vi "Read_Write_Plot_Setup.vi"(2 "Mode":enum16{"Load", "Save"}(ring), 3 "Setup filename":string, 4 "Cluster":T1={"Result files to read"=[], "Template"=path "", "Transpose"=FALSE, "Additional X Values"=[], "Additional Y Values"=[], "Ordinate"=0, "Absisca"=0, "Filter Array"=[0, 0, 0, 0, 0, 0], "color and symbol"=FALSE, "Output Filename"=path "", "Jpg Vi Name"="Intensity plot jpg.vi", "Intensity Plot?"=FALSE, "Multi Ordinate?"=FALSE, "Filter Bins 1"=[0], "Filter Bins 2"=[0], "Multi Ordinate"=[]} {"Filter Array" items=["Don't Filter", "Measurement Type", "Seconds Since 1904", "X [mm]", "Y [mm]", "Z [mm]", "U [ms-1] Raw", "U [ms-1]", "U/Uref", "V [ms-1]", "V/Uref", "W [ms-1]", "W/Uref", "u^2 [m2s-2] Raw", "u^2 [m2s-2]", "u^2/Ur^2", "v^2 [m2s-2] Raw", "v^2 [m2s-2]", "v^2/Ur^2", "w^2 [m2s-2] Raw", "w^2 [m2s-2]", "w^2/Ur^2", "uv [m2s-2] Raw", "uv [m2s-2]", "uv/Ur^2", "uw [m2s-2] Raw", "uw [m2s-2]", "uw/Ur^2", "Average Sampling Rate [Hz]", "Flow Measurement Time [mins]", "Tunnel Velocity Uref [ms-1]", "Measurement Record Date", "Measurement Record Time", "Original Results Folder", "Original Results Filename", "Original Results Raw Data File", "Comments", "Roughness Pattern", "Roughness Element", "Roughness Element Height (mm)", "Roughness Unit size", "Roughness Area Density (%)", "Roughness Elements In a Unit", "Roughness Baseboard Vertical Displacement (mm)", "A Tunnel Metadata Travers Origin X Offset", "XW Angle Psi 1", "XW Angle Psi 2", "Tutu & Chevray Error in uw Correlation", "XW (UW) Calibration Drift", "Reference Temperature Deg C"]; "Absisca" items=["Measurement Type", "Seconds Since 1904", "X [mm]", "Y [mm]", "Z [mm]", "U [ms-1] Raw", "U [ms-1]", "U/Uref", "V [ms-1]", "V/Uref", "W [ms-1]", "W/Uref", "u^2 [m2s-2] Raw", "u^2 [m2s-2]", "u^2/Ur^2", "v^2 [m2s-2] Raw", "v^2 [m2s-2]", "v^2/Ur^2", "w^2 [m2s-2] Raw", "w^2 [m2s-2]", "w^2/Ur^2", "uv [m2s-2] Raw", "uv [m2s-2]", "uv/Ur^2", "uw [m2s-2] Raw", "uw [m2s-2]", "uw/Ur^2", "Average Sampling Rate [Hz]", "Flow Measurement Time [mins]", "Tunnel Velocity Uref [ms-1]", "Measurement Record Date", "Measurement Record Time", "Original Results Folder", "Original Results Filename", "Original Results Raw Data File", "Comments", "Roughness Pattern", "Roughness Element", "Roughness Element Height (mm)", "Roughness Unit size", "Roughness Area Density (%)", "Roughness Elements In a Unit", "Roughness Baseboard Vertical Displacement (mm)", "A Tunnel Metadata Travers Origin X Offset", "XW Angle Psi 1", "XW Angle Psi 2", "Tutu & Chevray Error in uw Correlation", "XW (UW) Calibration Drift", "Reference Temperature Deg C"]; "Ordinate" items=["Measurement Type", "Seconds Since 1904", "X [mm]", "Y [mm]", "Z [mm]", "U [ms-1] Raw", "U [ms-1]", "U/Uref", "V [ms-1]", "V/Uref", "W [ms-1]", "W/Uref", "u^2 [m2s-2] Raw", "u^2 [m2s-2]", "u^2/Ur^2", "v^2 [m2s-2] Raw", "v^2 [m2s-2]", "v^2/Ur^2", "w^2 [m2s-2] Raw", "w^2 [m2s-2]", "w^2/Ur^2", "uv [m2s-2] Raw", "uv [m2s-2]", "uv/Ur^2", "uw [m2s-2] Raw", "uw [m2s-2]", "uw/Ur^2", "Average Sampling Rate [Hz]", "Flow Measurement Time [mins]", "Tunnel Velocity Uref [ms-1]", "Measurement Record Date", "Measurement Record Time", "Original Results Folder", "Original Results Filename", "Original Results Raw Data File", "Comments", "Roughness Pattern", "Roughness Element", "Roughness Element Height (mm)", "Roughness Unit size", "Roughness Area Density (%)", "Roughness Elements In a Unit", "Roughness Baseboard Vertical Displacement (mm)", "A Tunnel Metadata Travers Origin X Offset", "XW Angle Psi 1", "XW Angle Psi 2", "Tutu & Chevray Error in uw Correlation", "XW (UW) Calibration Drift", "Reference Temperature Deg C"]; "Additional Y Values" format="%.2f"; "Additional X Values" format="%.2f"}) -> (0 "OK?":bool, 1 "Cluster 2":T1={"Result files to read"=[], "Template"=path "", "Transpose"=FALSE, "Additional X Values"=[], "Additional Y Values"=[], "Ordinate"=0, "Absisca"=0, "Filter Array"=[0, 0, 0, 0, 0, 0], "color and symbol"=FALSE, "Output Filename"=path "", "Jpg Vi Name"="Intensity plot jpg.vi", "Intensity Plot?"=FALSE, "Multi Ordinate?"=FALSE, "Filter Bins 1"=[0], "Filter Bins 2"=[0], "Multi Ordinate"=[]} {"Filter Array" items=["Don't Filter", "Measurement Type", "Seconds Since 1904", "X [mm]", "Y [mm]", "Z [mm]", "U [ms-1] Raw", "U [ms-1]", "U/Uref", "V [ms-1]", "V/Uref", "W [ms-1]", "W/Uref", "u^2 [m2s-2] Raw", "u^2 [m2s-2]", "u^2/Ur^2", "v^2 [m2s-2] Raw", "v^2 [m2s-2]", "v^2/Ur^2", "w^2 [m2s-2] Raw", "w^2 [m2s-2]", "w^2/Ur^2", "uv [m2s-2] Raw", "uv [m2s-2]", "uv/Ur^2", "uw [m2s-2] Raw", "uw [m2s-2]", "uw/Ur^2", "Average Sampling Rate [Hz]", "Flow Measurement Time [mins]", "Tunnel Velocity Uref [ms-1]", "Measurement Record Date", "Measurement Record Time", "Original Results Folder", "Original Results Filename", "Original Results Raw Data File", "Comments", "Roughness Pattern", "Roughness Element", "Roughness Element Height (mm)", "Roughness Unit size", "Roughness Area Density (%)", "Roughness Elements In a Unit", "Roughness Baseboard Vertical Displacement (mm)", "A Tunnel Metadata Travers Origin X Offset", "XW Angle Psi 1", "XW Angle Psi 2", "Tutu & Chevray Error in uw Correlation", "XW (UW) Calibration Drift", "Reference Temperature Deg C"]; "Absisca" items=["Measurement Type", "Seconds Since 1904", "X [mm]", "Y [mm]", "Z [mm]", "U [ms-1] Raw", "U [ms-1]", "U/Uref", "V [ms-1]", "V/Uref", "W [ms-1]", "W/Uref", "u^2 [m2s-2] Raw", "u^2 [m2s-2]", "u^2/Ur^2", "v^2 [m2s-2] Raw", "v^2 [m2s-2]", "v^2/Ur^2", "w^2 [m2s-2] Raw", "w^2 [m2s-2]", "w^2/Ur^2", "uv [m2s-2] Raw", "uv [m2s-2]", "uv/Ur^2", "uw [m2s-2] Raw", "uw [m2s-2]", "uw/Ur^2", "Average Sampling Rate [Hz]", "Flow Measurement Time [mins]", "Tunnel Velocity Uref [ms-1]", "Measurement Record Date", "Measurement Record Time", "Original Results Folder", "Original Results Filename", "Original Results Raw Data File", "Comments", "Roughness Pattern", "Roughness Element", "Roughness Element Height (mm)", "Roughness Unit size", "Roughness Area Density (%)", "Roughness Elements In a Unit", "Roughness Baseboard Vertical Displacement (mm)", "A Tunnel Metadata Travers Origin X Offset", "XW Angle Psi 1", "XW Angle Psi 2", "Tutu & Chevray Error in uw Correlation", "XW (UW) Calibration Drift", "Reference Temperature Deg C"]; "Ordinate" items=["Measurement Type", "Seconds Since 1904", "X [mm]", "Y [mm]", "Z [mm]", "U [ms-1] Raw", "U [ms-1]", "U/Uref", "V [ms-1]", "V/Uref", "W [ms-1]", "W/Uref", "u^2 [m2s-2] Raw", "u^2 [m2s-2]", "u^2/Ur^2", "v^2 [m2s-2] Raw", "v^2 [m2s-2]", "v^2/Ur^2", "w^2 [m2s-2] Raw", "w^2 [m2s-2]", "w^2/Ur^2", "uv [m2s-2] Raw", "uv [m2s-2]", "uv/Ur^2", "uw [m2s-2] Raw", "uw [m2s-2]", "uw/Ur^2", "Average Sampling Rate [Hz]", "Flow Measurement Time [mins]", "Tunnel Velocity Uref [ms-1]", "Measurement Record Date", "Measurement Record Time", "Original Results Folder", "Original Results Filename", "Original Results Raw Data File", "Comments", "Roughness Pattern", "Roughness Element", "Roughness Element Height (mm)", "Roughness Unit size", "Roughness Area Density (%)", "Roughness Elements In a Unit", "Roughness Baseboard Vertical Displacement (mm)", "A Tunnel Metadata Travers Origin X Offset", "XW Angle Psi 1", "XW Angle Psi 2", "Tutu & Chevray Error in uw Correlation", "XW (UW) Calibration Drift", "Reference Temperature Deg C"]; "Additional Y Values" format="%.2f"; "Additional X Values" format="%.2f"})   [LabVIEW 2010]
uses:
  All_Setup.ctl
  File/Setup_Filetype.ctl
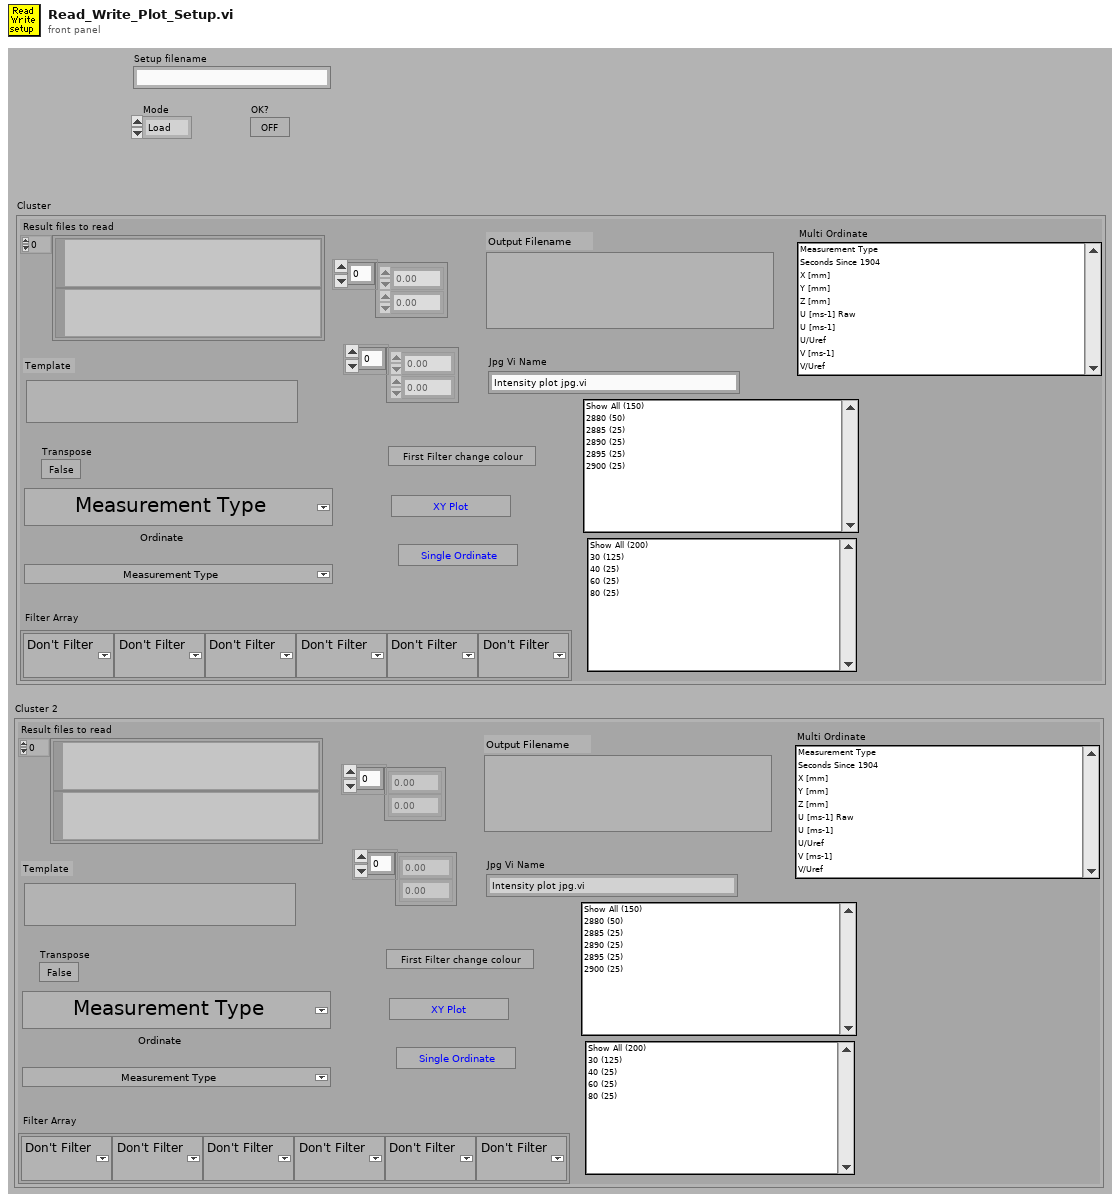
[diagram p1: front panel]
types:
  T1 = typedef "All_Setup.ctl" = cluster{"Result files to read":path[], "Template":path, "Transpose":bool, "Additional X Values":dbl[], "Additional Y Values":dbl[], "Ordinate":u16, "Absisca":u16, "Filter Array":u16[], "color and symbol":bool, "Output Filename":path, "Jpg Vi Name":string, "Intensity Plot?":bool, "Multi Ordinate?":bool, "Filter Bins 1":i32[], "Filter Bins 2":i32[], "Multi Ordinate":i32[]}
  T2 = typedef "Setup_Filetype.ctl" = enum16{"Measurement Setups", "Calibration Setups", "General", "Results File Plotter Setups", "Speed Calib Tweaks"}
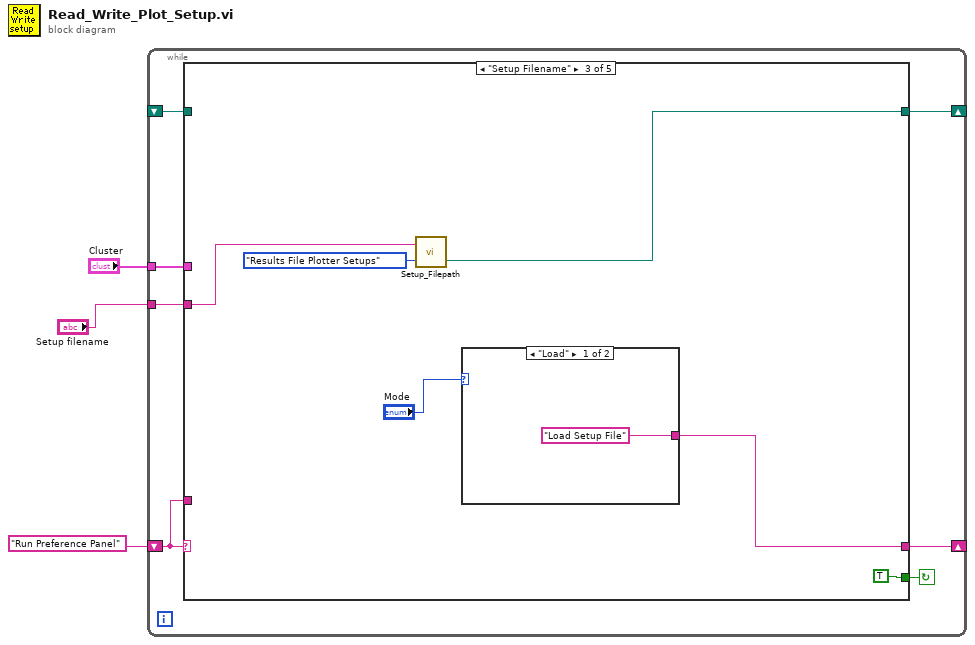
[diagram p0: block diagram]
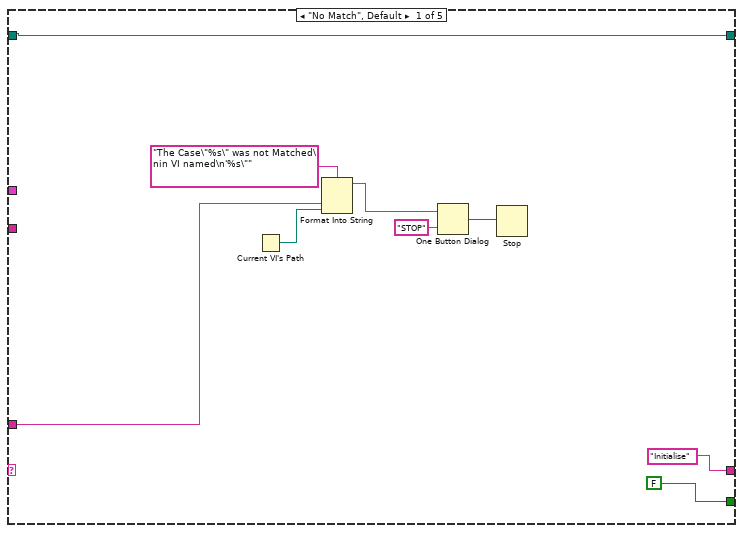
[diagram p2: hidden frame]
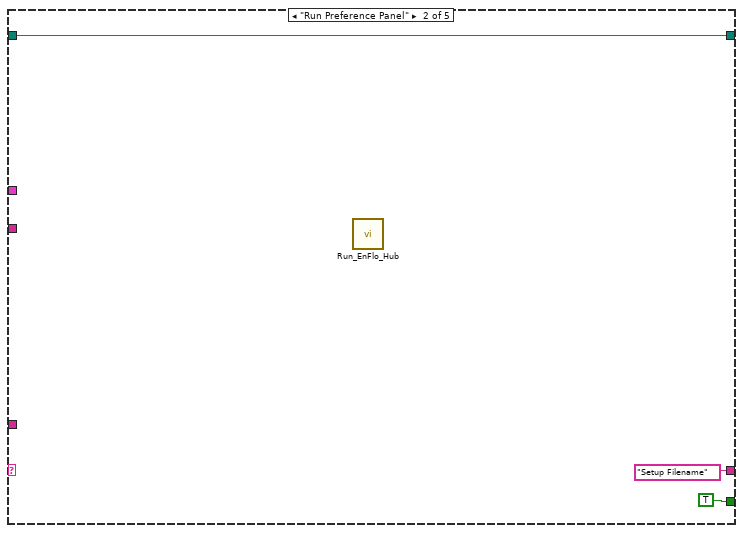
[diagram p3: hidden frame]
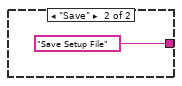
[diagram p4: hidden frame]
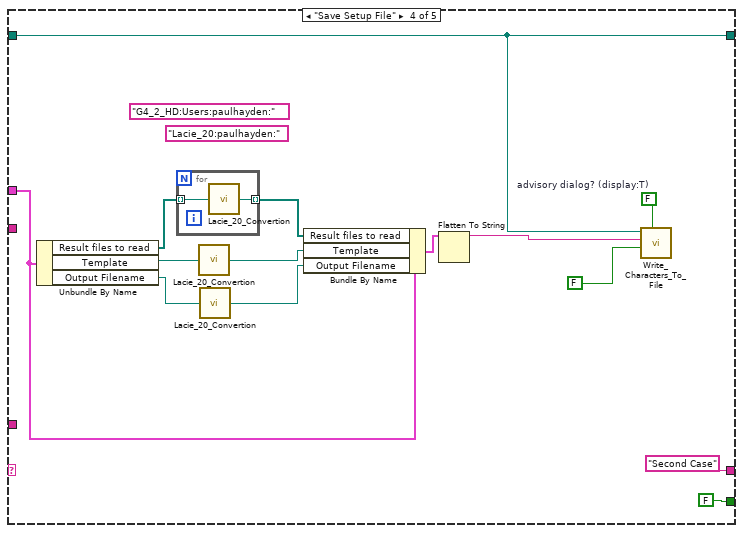
[diagram p5: hidden frame]
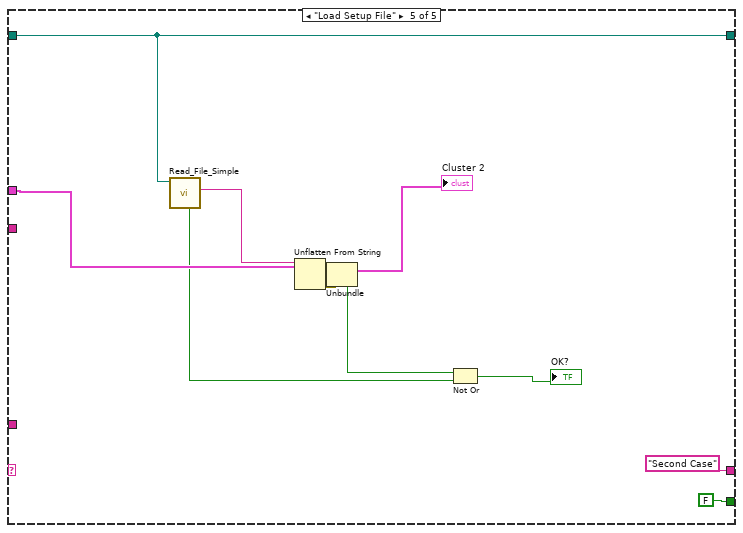
[diagram p6: hidden frame]
diagram:
  n1 = while {
    shift-left: "Run Preference Panel" -> [w8]
    shift-right: [w9] -> _
    shift-right: [w6] -> _
    shift-left: _ -> [w7]
    tunnel: "Cluster" -> [w5]
    tunnel: "Setup filename" -> [w4]
    stop <- w10 continue-if-true
    n2 = case shown="\"Setup Filename\"" w8 {
      tunnel: [FALSE TRUE TRUE FALSE FALSE] -> w10
      tunnel: ["Initialise" "Setup Filename" w26 "Second Case" "Second Case"] -> w9
      tunnel: w8 -> [w14 _ _ _ _]
      tunnel: w7 -> [w11 w20 _ w39 w48]
      tunnel: [w11 w20 w23 w39 w48] -> w6
      tunnel: w5 -> [_ _ _ w38 w53]
      tunnel: w4 -> [_ _ w24 _ _]
      frame "No Match", Default {
        n3 = Current VI's Path() -> (path=w13:path)
        n4 = Format Into String(format string="The Case\"%s\" was not Matched\nin VI named\n'%s\"" ("Format String"), w14, w13) -> (resulting string=w17:string)  [unwired: 2 in, 1 out]
        n5 = One Button Dialog(message=w17, button name ("OK")="STOP") -> (true=w15:bool)
        n6 = Stop(stop? (T)=w15) -> ()
      }
      frame "Run Preference Panel" {
        n7 = call "Run_EnFlo_Hub.vi"() -> ()  [unwired: 8 out]
      }
      frame "Setup Filename" {
        n8 = call "Setup_Filepath.vi"("Setup File Type"=Setup_Filetype."Results File Plotter Setups", "Filename in"=w24) -> ("Filename Out"=w23:path)  [unwired: 1 out]
        n9 = case shown="\"Load\"" "Mode" {
          tunnel: ["Load Setup File" "Save Setup File"] -> w26
          frame "Load" {
          }
          frame "Save" {
          }
        }
      }
      frame "Save Setup File" {
        (unwired) "Lacie_20:paulhayden:"
        (unwired) "G4_2_HD:Users:paulhayden:"
        w40 = FALSE  # advisory dialog? (display:T)
        n10 = Unbundle By Name(w38) -> ("Result files to read"=w34:path[], "Template"=w33:path, "Output Filename"=w32:path)
        n11 = for {
          tunnel: [w46] -> w35 mode=indexing
          tunnel: w34 -> [w45] mode=indexing
          n12 = call "Lacie_20_Convertion.vi"("Path"=w45) -> ("Path 2"=w46:path)
        }
        n13 = call "Lacie_20_Convertion.vi"("Path"=w33) -> ("Path 2"=w36:path)
        n14 = call "Lacie_20_Convertion.vi"("Path"=w32) -> ("Path 2"=w37:path)
        n15 = Bundle By Name(cluster=w38, "Result files to read"=w35, "Template"=w36, "Output Filename"=w37) -> (w31:T1)
        n16 = Flatten To String(anything=w31) -> (data string=w42:string)  [unwired: 1 in, 4 out]
        n17 = call "Write_Characters_To_File.vi"("file path (dialog if empty)"=w39, "advisory dialog? (display:T)"=w40, "character string"=w42, "append to file? (new file:F)"=FALSE) -> ()  [unwired: 1 in, 4 out]
      }
      frame "Load Setup File" {
        n18 = call "Read_File_Simple.vi"("Filename"=w48) -> ("Error?"=w50:bool, "string"=w54:string)  [unwired: 2 in, 6 out]
        n19 = Unflatten From String(type=w53, binary string=w54) -> (value=→"Cluster 2":T1, error out=w47:errorcluster)  [unwired: 1 in, 3 out]
        n20 = Unbundle(w47) -> ("status"=w51:bool)  [unwired: 2 out]
        n21 = Not Or(1:w50, 2:w51) -> (0:→"OK?":bool)
      }
    }
  }
